vi "LJM_eWriteAddresses.vi"(0 "Handle In":i32, 1 "NumFrames":i32, 5 "aAddresses":i32[](array[numeric]), 7 "aTypes":i32[](array[numeric]), 9 "aValues":dbl[](array[numeric]) format="%.2f", 11 "error in":errorcluster) -> (4 "Handle Out":i32, 14 "ErrorAddress":i32, 15 "error out":errorcluster)   [LabVIEW 2017]
uses:
  labjackm.dll
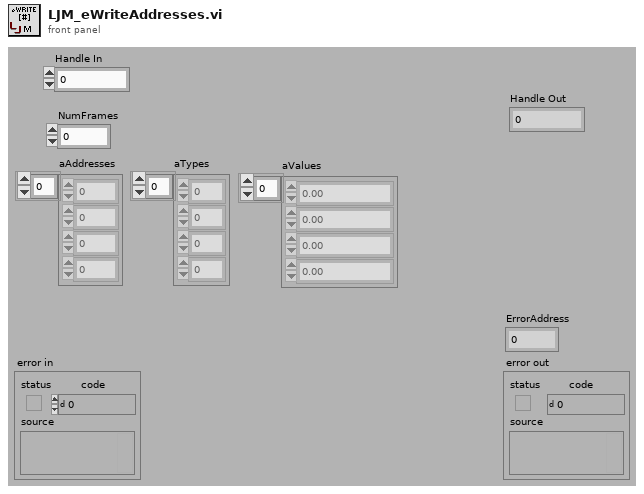
[diagram p1: front panel]
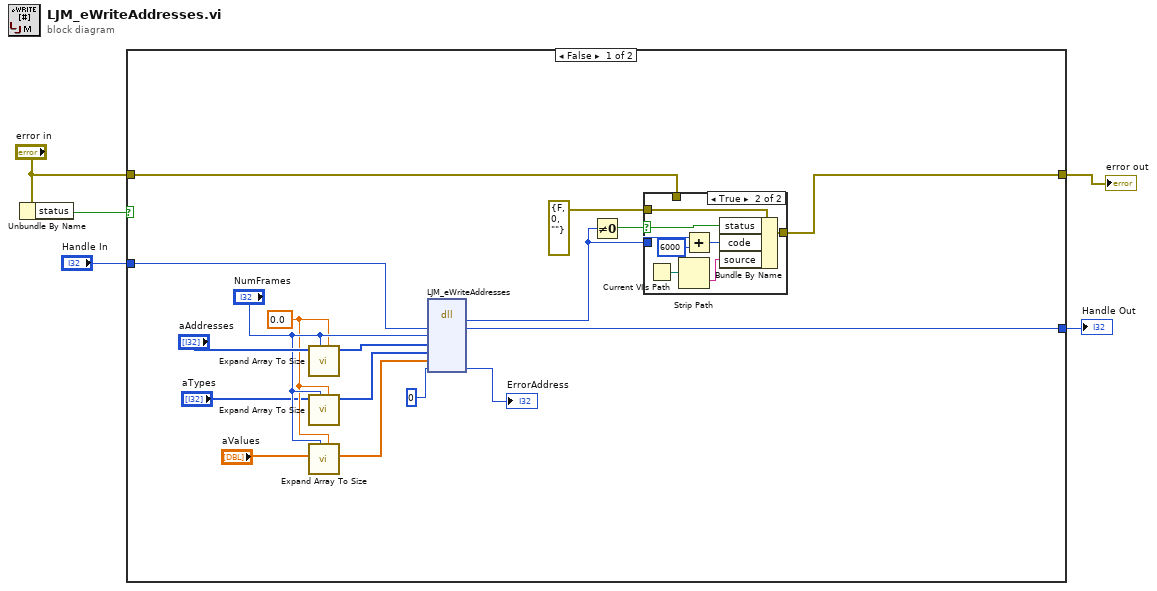
[diagram p0: block diagram]
diagram:
  n1 = Unbundle By Name("error in") -> ("status"=w5:bool)
  n2 = case shown="False" w5 {
    tunnel: "error in" -> [w19 w33]
    tunnel: [w18 w33] -> w3
    tunnel: "Handle In" -> [w7 w32]
    tunnel: [w6 w32] -> w1
    frame False {
      w14 = 0.0 ("Default Value")
      n3 = call <userlib>:"Expand Array To Size.vi"("Default Value"=w14, "# Elements"="NumFrames", "I32 Array In"="aAddresses") -> ("I32 Array Out"=w16:i32[])  [unwired: 4 in, 4 out]
      n4 = call <userlib>:"Expand Array To Size.vi"("Default Value"=w14, "# Elements"="NumFrames", "I32 Array In"="aTypes") -> ("I32 Array Out"=w12:i32[])  [unwired: 4 in, 4 out]
      n5 = call <userlib>:"Expand Array To Size.vi"("Default Value"=w14, "# Elements"="NumFrames", "DBL Array In"="aValues") -> ("DBL Array Out"=w11:dbl[])  [unwired: 4 in, 4 out]
      n6 = dll-call lib="labjackm.dll" fn="LJM_eWriteAddresses"("Handle"=w7, "NumFrames"="NumFrames", "aAddresses"=w16, "aTypes"=w12, "aValues"=w11, "ErrorFrame"=u32 0) -> (w22:i32, "Handle"=w6:i32, "ErrorFrame"=→"ErrorAddress":i32)  [unwired: 7 in, 2 out]
      n7 = Not Equal To 0?(x=w22) -> (x != 0?=w21:bool)
      n8 = case shown="True" w21 {
        selector: w21 -> [_ w30]
        tunnel: [w23 w31] -> w18
        tunnel: errorcluster {"status"=FALSE, "code"=0, "source"=""} ("error IO") -> [_ w29]
        tunnel: w22 -> [_ w25]
        tunnel: w19 -> [w23 _]
        frame False {
        }
        frame True {
          n9 = Current VI's Path() -> (path=w27:path)
          n10 = Strip Path(path=w27) -> (name=w28:string)  [unwired: 1 out]
          n11 = Add(x=w25, y=6000) -> (x+y=w26:i32)
          n12 = Bundle By Name(cluster=w29, "status"=w30, "code"=w26, "source"=w28) -> (w31:errorcluster)
        }
      }
    }
    frame True {
    }
  }
  "error out" <- w3
  "Handle Out" <- w1
